vi "首页_古田户外.vi"() -> ()   [LabVIEW 2016]
uses:
  <vilib>/Utility/miscctls.llb/LVPointTypeDef.ctl
  <vilib>/Utility/sysdir.llb/System Directory Type.ctl
  <vilib>/addons/database/_DB Variant To Data/Database Variant To Data.xnode
  PLC/PLC.lvlib
panel:
  out "小项目框 9":T1(xcontrol)
  out "小项目框 8":T1(xcontrol)
  out "小项目框 7":T1(xcontrol)
  out "小项目框 6":T1(xcontrol)
  out "小项目框 5":T1(xcontrol)
  out "小项目框":T1(xcontrol)
  out "湿度":string="75.5 %"
  out "室温":string="25.8 ℃"
  out "小项目框 4":T1(xcontrol)
  out "小项目框 3":T1(xcontrol)
  out "小项目框 2":T1(xcontrol)
  # "湿度:"
  # "室温:"
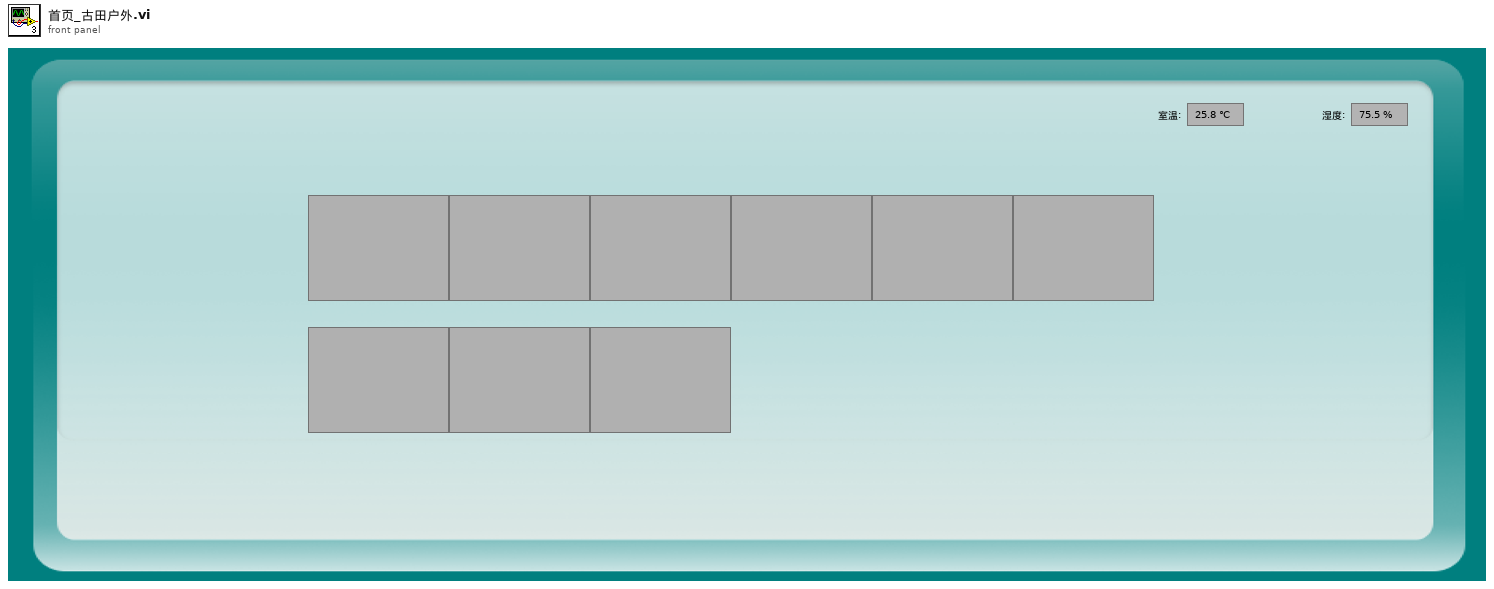
[diagram p1: front panel]
types:
  T1 = cluster{"中文项目名称":string, "英文项目名称":string, "单位":string, "浓度值":sgl}
  T2 = typedef "System Directory Type.ctl" = i32
  T3 = typedef "LVPointTypeDef.ctl" = cluster{"Horizontal":i16, "Vertical":i16}
  T4 = cluster{"AD0":sgl, "AD1":sgl, "AD2":sgl, "AD3":sgl, "AD4":sgl, "AD5":sgl}
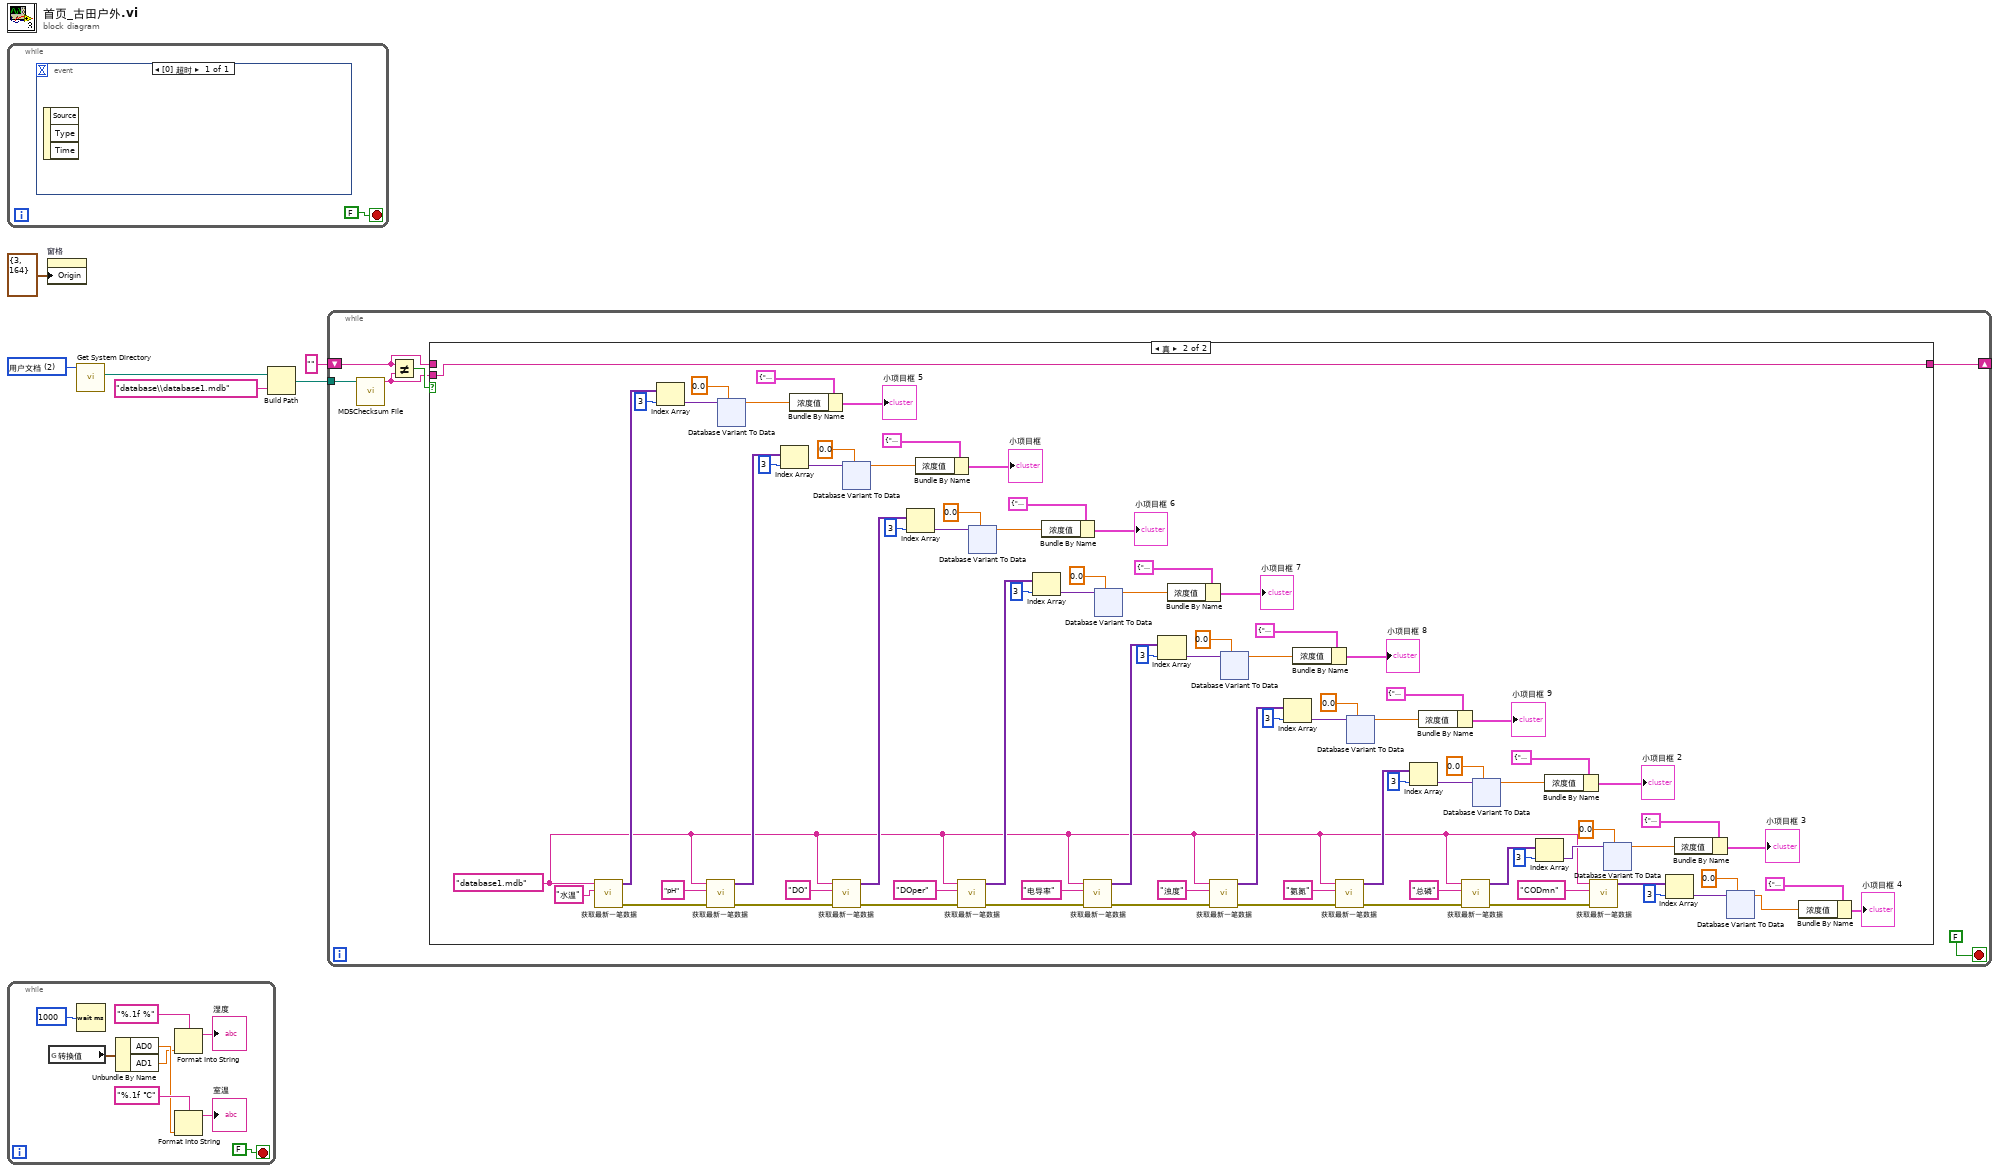
[diagram p0: block diagram]
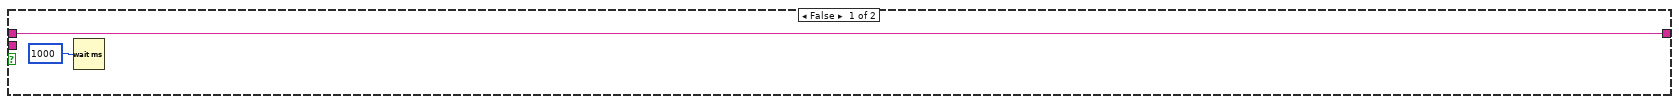
[diagram p2: hidden frame]
diagram:
  w5 = T2 2 items=["用户目录"=0, "用户桌面"=1, "用户文档"=2, "用户应用程序数据"=3, "用户设置"=4, "用户临时目录"=5, "公共文档"=6, "公共应用程序数据"=7, "公共设置"=8, "公共缓存"=13, "系统核心库"=9, "系统安装库"=10, "应用程序文件"=11, "启动盘根目录"=12] ("system directory type")
  n1 = while {
    stop <- FALSE stop-if-true
    n2 = event shown="[0] 超时" {
      selector: _ -> [_]
      dyn-events: _ -> [_]
      timeout: _ -> [_]
      event Timeout {
        n3 = event-data() -> ()  [unwired: 1 in, 3 out]
      }
    }
  }
  n4 = while {
    stop <- FALSE stop-if-true
    n5 = global read "采配水全局变量.vi" "转换值"() -> (w14:T4)
    n6 = Wait (ms)(milliseconds to wait=u32 1000 ("等待时间（毫秒）")) -> ()  [unwired: 1 out]
    n7 = Unbundle By Name(w14) -> ("AD0"=w9:sgl, "AD1"=w8:sgl)
    n8 = Format Into String(format string="%.1f %" ("格式字符串"), w8) -> (resulting string=→"湿度":string)  [unwired: 2 in, 1 out]
    n9 = Format Into String(format string="%.1f ℃" ("格式字符串"), w9) -> (resulting string=→"室温":string)  [unwired: 2 in, 1 out]
  }
  n10 = property on="窗格" class="Pane"("Origin"=T3 {"Horizontal"=3, "Vertical"=164} ("原点")) -> ()  [unwired: 2 in, 2 out]
  n11 = call <vilib>:"Get System Directory.vi"("system directory type"=w5) -> ("system directory"=w4:path)  [unwired: 10 in]
  n12 = Build Path(base path=w4, name or relative path="database\\database1.mdb" ("名称或相对路径")) -> (appended path=w2:path)
  n13 = while {
    tunnel: w2 -> [w22]
    shift-right: [w19] -> _
    shift-left: "" ("MD5 message-digest") -> [w18]
    stop <- FALSE stop-if-true
    n14 = call <vilib>:"MD5Checksum File.vi"("Path"=w22) -> ("MD5 message-digest"=w20:string)  [unwired: 9 in, 1 out]
    n15 = Not Equal?(x=w18, y=w20) -> (x != y?=w21:bool)
    n16 = case shown="真" w21 {
      tunnel: w20 -> [_ w106]
      tunnel: [w24 w106] -> w19
      tunnel: w18 -> [w24 _]
      frame False {
        n17 = Wait (ms)(milliseconds to wait=u32 1000 ("等待时间（毫秒）")) -> ()  [unwired: 1 out]
      }
      frame True {
        w30 = "database1.mdb" ("名称或相对路径")
        n18 = call "获取最新一笔数据.vi"("table"="水温", "database"=w30) -> ("error out"=w70:errorcluster, "子数组"=w36:variant[])  [unwired: 8 in]
        n19 = Index Array(array=w36, index=3 ("索引")) -> (element=w59:variant)
        n20 = call "获取最新一笔数据.vi"("error in (no error)"=w70, "table"="pH", "database"=w30) -> ("error out"=w69:errorcluster, "子数组"=w95:variant[])  [unwired: 7 in]
        n21 = xnode "Database Variant To Data"("database variant"=w59, "type"=0.0) -> ("data"=w61:dbl)  [unwired: 1 in, 1 out]
        n22 = Index Array(array=w95, index=3 ("索引")) -> (element=w78:variant)
        n23 = Bundle By Name(cluster=T1 {"中文项目名称"="水温", "英文项目名称"="T", "单位"="℃", "浓度值"=0.0} ("小项目框 9"), "浓度值"=w61) -> (→"小项目框 5":T1)
        n24 = call "获取最新一笔数据.vi"("error in (no error)"=w69, "table"="DO", "database"=w30) -> ("error out"=w67:errorcluster, "子数组"=w35:variant[])  [unwired: 7 in]
        n25 = xnode "Database Variant To Data"("database variant"=w78, "type"=0.0) -> ("data"=w76:dbl)  [unwired: 1 in, 1 out]
        n26 = Index Array(array=w35, index=3 ("索引")) -> (element=w54:variant)
        n27 = Bundle By Name(cluster=T1 {"中文项目名称"="酸碱度", "英文项目名称"="pH", "单位"="", "浓度值"=0.0} ("小项目框 9"), "浓度值"=w76) -> (→"小项目框":T1)
        n28 = call "获取最新一笔数据.vi"("error in (no error)"=w67, "table"="DOper", "database"=w30) -> ("error out"=w65:errorcluster, "子数组"=w34:variant[])  [unwired: 7 in]
        n29 = xnode "Database Variant To Data"("database variant"=w54, "type"=0.0) -> ("data"=w52:dbl)  [unwired: 1 in, 1 out]
        n30 = Index Array(array=w34, index=3 ("索引")) -> (element=w49:variant)
        n31 = Bundle By Name(cluster=T1 {"中文项目名称"="溶解氧", "英文项目名称"="DO", "单位"="mg/L", "浓度值"=0.0} ("小项目框 9"), "浓度值"=w52) -> (→"小项目框 6":T1)
        n32 = call "获取最新一笔数据.vi"("error in (no error)"=w65, "table"="电导率", "database"=w30) -> ("error out"=w63:errorcluster, "子数组"=w33:variant[])  [unwired: 7 in]
        n33 = xnode "Database Variant To Data"("database variant"=w49, "type"=0.0) -> ("data"=w51:dbl)  [unwired: 1 in, 1 out]
        n34 = Index Array(array=w33, index=3 ("索引")) -> (element=w44:variant)
        n35 = Bundle By Name(cluster=T1 {"中文项目名称"="溶解氧%", "英文项目名称"="DO%", "单位"="%", "浓度值"=0.0} ("小项目框 9"), "浓度值"=w51) -> (→"小项目框 7":T1)
        n36 = call "获取最新一笔数据.vi"("error in (no error)"=w63, "table"="浊度", "database"=w30) -> ("error out"=w62:errorcluster, "子数组"=w32:variant[])  [unwired: 7 in]
        n37 = xnode "Database Variant To Data"("database variant"=w44, "type"=0.0) -> ("data"=w42:dbl)  [unwired: 1 in, 1 out]
        n38 = Index Array(array=w32, index=3 ("索引")) -> (element=w39:variant)
        n39 = Bundle By Name(cluster=T1 {"中文项目名称"="电导率", "英文项目名称"="Cond", "单位"="uS/cm", "浓度值"=0.0} ("小项目框 9"), "浓度值"=w42) -> (→"小项目框 8":T1)
        n40 = call "获取最新一笔数据.vi"("error in (no error)"=w62, "table"="氨氮", "database"=w30) -> ("error out"=w104:errorcluster, "子数组"=w90:variant[])  [unwired: 7 in]
        n41 = xnode "Database Variant To Data"("database variant"=w39, "type"=0.0) -> ("data"=w41:dbl)  [unwired: 1 in, 1 out]
        n42 = Index Array(array=w90, index=3 ("索引")) -> (element=w84:variant)
        n43 = Bundle By Name(cluster=T1 {"中文项目名称"="浊度", "英文项目名称"="Turb", "单位"="NTU", "浓度值"=0.0} ("小项目框 9"), "浓度值"=w41) -> (→"小项目框 9":T1)
        n44 = call "获取最新一笔数据.vi"("error in (no error)"=w104, "table"="总磷", "database"=w30) -> ("error out"=w72:errorcluster, "子数组"=w85:variant[])  [unwired: 7 in]
        n45 = xnode "Database Variant To Data"("database variant"=w84, "type"=0.0) -> ("data"=w82:dbl)  [unwired: 1 in, 1 out]
        n46 = Index Array(array=w85, index=3 ("索引")) -> (element=w81:variant)
        n47 = Bundle By Name(cluster=T1 {"中文项目名称"="氨氮", "英文项目名称"="NH3-N", "单位"="mg/L", "浓度值"=0.0} ("小项目框 9"), "浓度值"=w82) -> (→"小项目框 2":T1)
        n48 = call "获取最新一笔数据.vi"("error in (no error)"=w72, "table"="CODmn", "database"=w30) -> ("子数组"=w98:variant[])  [unwired: 7 in, 1 out]
        n49 = xnode "Database Variant To Data"("database variant"=w81, "type"=0.0) -> ("data"=w79:dbl)  [unwired: 1 in, 1 out]
        n50 = Index Array(array=w98, index=3 ("索引")) -> (element=w75:variant)
        n51 = Bundle By Name(cluster=T1 {"中文项目名称"="总磷", "英文项目名称"="TP", "单位"="mg/L", "浓度值"=0.0} ("小项目框 9"), "浓度值"=w79) -> (→"小项目框 3":T1)
        n52 = xnode "Database Variant To Data"("database variant"=w75, "type"=0.0) -> ("data"=w73:dbl)  [unwired: 1 in, 1 out]
        n53 = Bundle By Name(cluster=T1 {"中文项目名称"="高锰酸盐指数", "英文项目名称"="CODmn", "单位"="mg/L", "浓度值"=0.0} ("小项目框 9"), "浓度值"=w73) -> (→"小项目框 4":T1)
      }
    }
  }
